vi "PathPlanner_FieldUtil_FlipFieldRotation.vi"(11 "rotation":T1={"VALUE"=0.0, "COS"=1.0, "SIN"=0.0} {"SIN" format="%13.4f"; "COS" format="%13.4f"; "VALUE" format="%13.4f"}) -> (3 "flippedRotation":T1={"VALUE"=0.0, "COS"=1.0, "SIN"=0.0} {"SIN" format="%13.4f"; "COS" format="%13.4f"; "VALUE" format="%13.4f"})   [LabVIEW 2019, in "PathPlanner24.lvlib"]
doc: "Flip a field rotation\n\nInput:\n -- FieldRotation\n\nOutputs:\n -- FlippedFieldRotation"
uses:
  PathPlanner24.lvlib
  <vilib>/Rock Robotics/WPI/ThirdParty/JAS_Junk/TrajLib/TypeDef/ROTATION2D.ctl
  <vilib>/Rock Robotics/WPI/ThirdParty/JAS_Junk/TrajLib/Rotation2d_UnaryMinus.vi
  <vilib>/Rock Robotics/WPI/ThirdParty/JAS_Junk/TrajLib/Rotation2d_RotateBy.vi
  <vilib>/Rock Robotics/WPI/ThirdParty/JAS_Junk/TrajLib/Rotation2d_CreateXY.vi
  <vilib>/Rock Robotics/WPI/ThirdParty/JAS_Junk/TrajLib/Util_CalcDist.vi
  <vilib>/Rock Robotics/WPI/ThirdParty/JAS_Junk/TrajLib/Trajectory_Library.lvlib
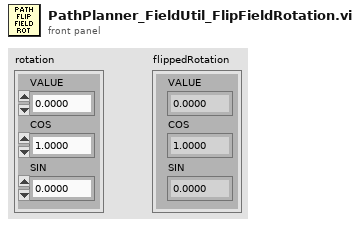
[diagram p1: front panel]
types:
  T1 = typedef "Trajectory_Library.lvlib/ROTATION2D.ctl" = cluster{"VALUE":dbl, "COS":dbl, "SIN":dbl}
  T2 = typedef "PathPlanner24.lvlib/PathPlanner_FieldSymmetry_ENUM.ctl" = enum16{"kRotational", "kMirrored"}
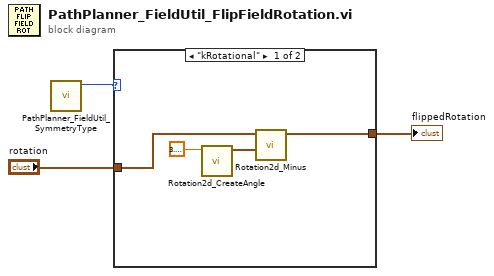
[diagram p0: block diagram]
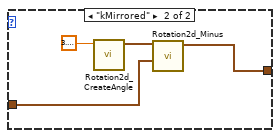
[diagram p2: hidden frame]
diagram:
  n1 = call "PathPlanner_FieldUtil_SymmetryType.vi"() -> ("PathPlanner_FieldSymmetry"=w3:T2)  [unwired: 11 in]
  n2 = case shown="\"kRotational\"" w3 {
    tunnel: "rotation" -> [w6 w9]
    tunnel: [w4 w8] -> w1
    frame "kRotational" {
      n3 = call <vilib>:"Rotation2d_CreateAngle.vi"("Angle"=3.141592653589793) -> ("ROTATION"=w5:T1)  [unwired: 10 in]
      n4 = call <vilib>:"Rotation2d_Minus.vi"("other ROTATION"=w5, "in ROTATION"=w6) -> ("out ROTATION"=w4:T1)  [unwired: 9 in]
    }
    frame "kMirrored" {
      n5 = call <vilib>:"Rotation2d_CreateAngle.vi"("Angle"=3.141592653589793) -> ("ROTATION"=w10:T1)  [unwired: 10 in]
      n6 = call <vilib>:"Rotation2d_Minus.vi"("other ROTATION"=w9, "in ROTATION"=w10) -> ("out ROTATION"=w8:T1)  [unwired: 9 in]
    }
  }
  "flippedRotation" <- w1
